vi "Read Temperatures.vi"(8 "error in (no error)":errorcluster, 11 "gData in":refnum<class "gData.lvclass">) -> (0 "error out":errorcluster, 2 "Temperatures":T1, 3 "gData out":refnum<class "gData.lvclass">)   [LabVIEW 2016, in "gData.lvclass"]
uses:
  gData.lvclass
  gData.lvclass/gData.ctl
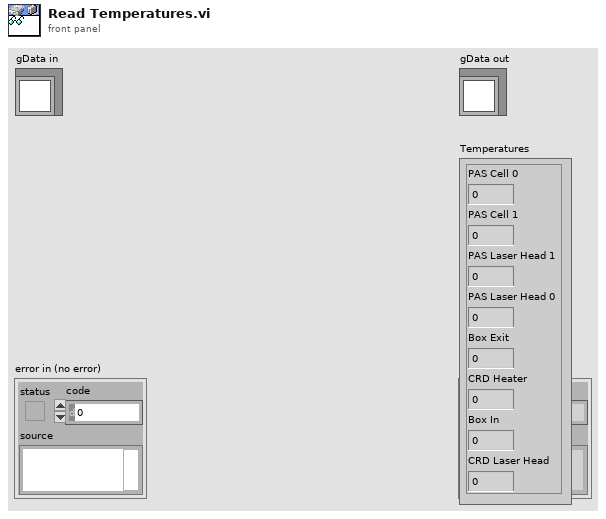
[diagram p1: front panel]
types:
  T1 = cluster{"PAS Cell 0":dbl, "PAS Cell 1":dbl, "PAS Laser Head 1":dbl, "PAS Laser Head 0":dbl, "Box Exit":dbl, "CRD Heater":dbl, "Box In":dbl, "CRD Laser Head":dbl}
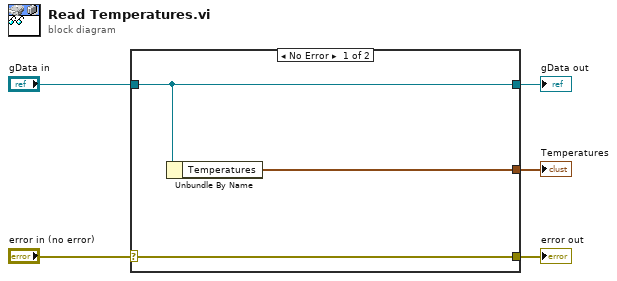
[diagram p0: block diagram]
diagram:
  n1 = case shown="No Error" "error in (no error)" {
    selector: "error in (no error)" -> [w8 w9]
    tunnel: [w8 w9] -> w4
    tunnel: [w7 w10] -> w2
    tunnel: "gData in" -> [w7 w10]
    tunnel: [w6 _] -> w1
    frame No Error {
      n2 = Unbundle By Name(w7) -> ("Temperatures"=w6:T1)
    }
    frame Error {
    }
  }
  "error out" <- w4
  "gData out" <- w2
  "Temperatures" <- w1
